vi "Modify Parent VI Title.vi"(0 "Title":string) -> ()   [LabVIEW 2021, in "EDT VIE.lvlib"]
uses:
  EDT VIE.lvlib
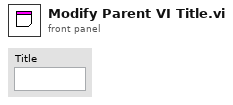
[diagram p1: front panel]
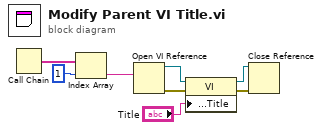
[diagram p0: block diagram]
diagram:
  n1 = Call Chain() -> (call chain=w8:string[])
  n2 = Index Array(array=w8, index=1) -> (element=w6:string)
  n3 = Open VI Reference(vi path=w6) -> (vi reference=w5:refnum<vi>, error out=w4:errorcluster)  [unwired: 5 in]
  n4 = property class="VI"(reference=w5, error in=w4, "Front Panel.Title"="Title") -> (reference out=w1:refnum<vi>, error out=w2:errorcluster)
  n5 = Close Reference(reference=w1, error in (no error)=w2) -> ()  [unwired: 1 out]
